vi "one_minus.vi"(4 "x":dbl) -> (1 "1-x":dbl)   [LabVIEW 2010]
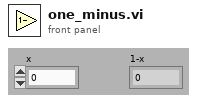
[diagram p1: front panel]
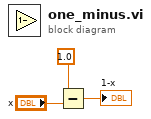
[diagram p0: block diagram]
diagram:
  n1 = Subtract(x=1.0, y="x") -> (x-y=→"1-x":dbl)
